vi "RSZVB Set Start To Marker.vi"(8 "error in (no error)":errorcluster {"code" format="%.0x"}, 9 "Marker (1)":i32=1, 10 "Channel (Trace) (1)":i32=1, 11 "VISA session":refnum<visa-resource-name>) -> (0 "error out":errorcluster {"code" format="%.0x"}, 3 "dup VISA session":refnum<visa-resource-name>)   [LabVIEW 2011]
doc: "This VI sets the beginning (start) of the sweep range equal to the stimulus value of the marker <Mk> on trace no. <Ch/Tr>.\n\nRemote-control command(s):\nCALCulate<Ch/Tr>:MARKer<Mk>:FUNCtion:STARt"
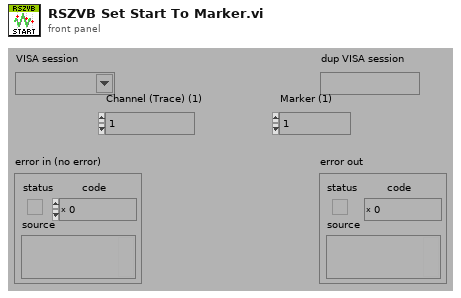
[diagram p1: front panel]
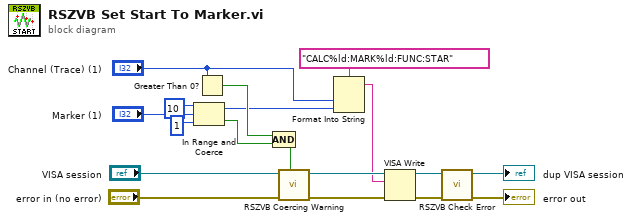
[diagram p0: block diagram]
diagram:
  n1 = In Range and Coerce(upper limit=10, x="Marker (1)", lower limit=1) -> (coerced(x)=w1:i32, In Range?=w10:bool)
  n2 = Greater Than 0?(x="Channel (Trace) (1)") -> (x > 0?=w13:bool)
  n3 = Compound Arithmetic op=AND(w13, w10) -> (w9:bool)
  n4 = call "RSZVB Coercing Warning.vi"("In Range?"=w9, "error in (no error)"="error in (no error)", "VISA session"="VISA session") -> ("error out"=w17:errorcluster, "dup VISA session"=w18:refnum<visa-resource-name>)  [unwired: 7 in]
  n5 = Format Into String(format string="CALC%ld:MARK%ld:FUNC:STAR", "Channel (Trace) (1)", w1) -> (resulting string=w8:string)  [unwired: 2 in, 1 out]
  n6 = VISA Write(VISA resource name=w18, write buffer=w8, error in (no error)=w17) -> (VISA resource name out=w15:refnum<visa-resource-name>, error out=w16:errorcluster)  [unwired: 1 out]
  n7 = call "RSZVB Check Error.vi"("error in (no error)"=w16, "VISA session"=w15) -> ("error out"=→"error out":errorcluster, "dup VISA session"=→"dup VISA session":refnum<visa-resource-name>)  [unwired: 8 in]
